vi "GlobalStop.vi"() -> ()   [LabVIEW 2020]
doc: "Global variable used to all program loop stop."
panel:
  in  "Stop":bool
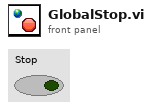
[diagram p1: front panel]
diagram:
